vi "TCP Status Check.vi"(8 "error in":errorcluster, 10 "Clients":refnum<k5>[](array[refnum]), 11 "listener":refnum<k5>) -> (0 "no error":errorcluster, 2 "Clients":refnum<k5>[](array[refnum]), 3 "Send Data":bool)   [LabVIEW 2020, in "TCP Server.lvlib"]
uses:
  TCP Server.lvlib
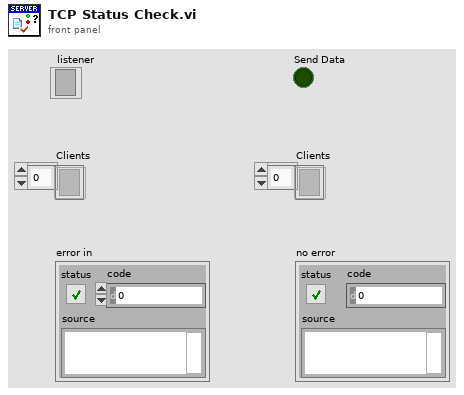
[diagram p1: front panel]
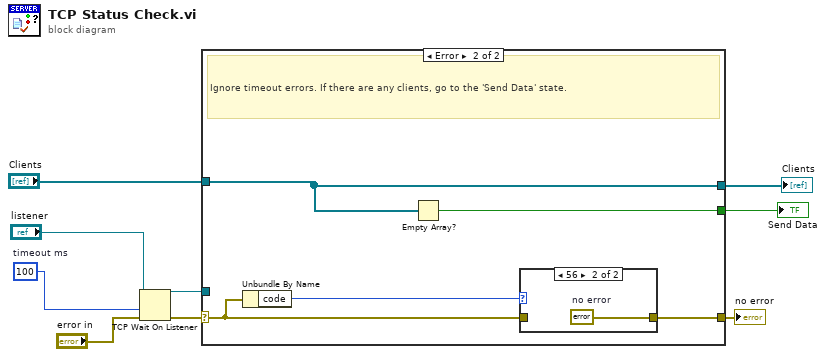
[diagram p0: block diagram]
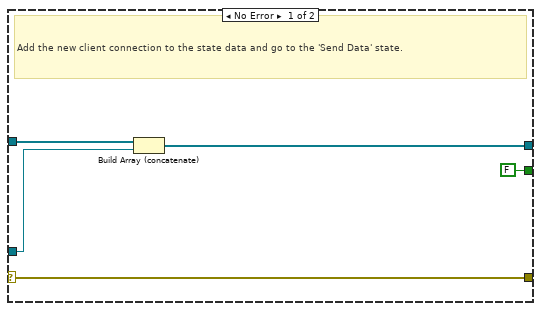
[diagram p2: hidden frame]
diagram:
  w7 = 100  # timeout ms
  n1 = TCP Wait On Listener(8:"error in", 9:w7, 11:"listener") -> (0:w8:errorcluster, 4:w9:refnum<k5>)  [unwired: 4 out]
  n2 = case shown="Error" w8 {
    selector: w8 -> [w14 w19]
    tunnel: w9 -> [w13 _]
    tunnel: [w14 w17] -> w3
    tunnel: "Clients" -> [w12 w16]
    tunnel: [w11 w16] -> w5
    tunnel: [FALSE ("empty?") w15] -> w4
    frame No Error {
      # "Add the new client connection to the state data and go to the 'Send Data' state."
      n3 = Build Array (concatenate)(w12, w13) -> (w11:refnum<k5>[])
    }
    frame Error {
      # "Ignore timeout errors. If there are any clients, go to the 'Send Data' state."
      n4 = Unbundle By Name(w19) -> ("code"=w18:i32)
      n5 = Empty Array?(array=w16) -> (empty?=w15:bool)
      n6 = case shown="56" w18 {
        tunnel: w19 -> [w20 _]
        tunnel: [w20 w21] -> w17
        frame Default {
        }
        frame 56 {
          w21 = errorcluster {"status"=FALSE, "code"=0, "source"=""}  # no error
        }
      }
    }
  }
  "Clients" <- w5
  "Send Data" <- w4
  "no error" <- w3
